vi "sensor cmd user calibration data blob.vi"(9 "dest_length":i32, 10 "dest":string, 11 "dev_handle":u32) -> (1 "function return":i32, 2 "dest out":string, 3 "dev_handle out":u32)   [LabVIEW 2019, in "apdm.lvlib"]
doc: "APDM_EXPORT int apdm_sensor_cmd_user_calibration_data_blob(apdm_device_handle_t dev_handle, uint8_t *dest, const int dest_length);"
uses:
  apdm.lvlib
  Lee Lab/CP FES Walking 2018/Code/Working/LabVIEW/apdm.dll
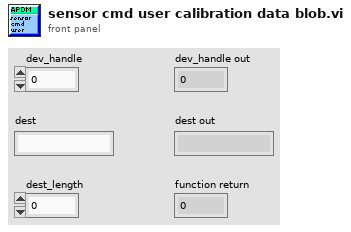
[diagram p1: front panel]
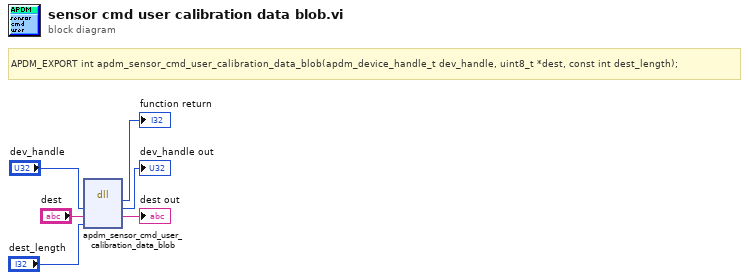
[diagram p0: block diagram]
diagram:
  # "APDM_EXPORT int apdm_sensor_cmd_user_calibration_data_blob(apdm_device_handle_t dev_handle, uint8_t *dest, const int dest_length);"
  n1 = dll-call lib="C:/Users/jfalesi/Dropbox/Lee Lab/CP FES Walking 2018/Code/Working/LabVIEW/apdm.*" fn="apdm_sensor_cmd_user_calibration_data_blob"("dev_handle"="dev_handle", "dest"="dest", "dest_length"="dest_length") -> (→"function return":i32, "dev_handle"=→"dev_handle out":u32, "dest"=→"dest out":string)  [unwired: 4 in, 2 out]
